vi "Parse rules to postfix.vi"(11 "String":string) -> (3 "Array":T1[](array[typedef]))   [LabVIEW 2019, in "LSS.lvlib"]
doc: "To allow the property control engine to fire events based on multiple conditions, a posfix calculator is used to evaluate the condions. This VI turns the Infix string based by the user to a postfix format that the control engine can read.\n\n<b>Inputs:</b>\n<b>String</b> - Infix string that must be parsed to postfix notation.\n<b>Error In</b> - Standard Error In terminal.\n\n<b>Outputs:</b>\n<b>Postfix</b> - Postfix notation of the input string.\n<b>Error Out</b> - Standard Error out terminal."
uses:
  LSS.lvlib
  Controls/Criteria.ctl
  Controls/Comparison Types.ctl
  <vilib>/regexp/Match Regular Expression.xnode
panel:
  out "Postfix":string[](array[string])
  out "error out":errorcluster
  out "Infix":string[](array[string])
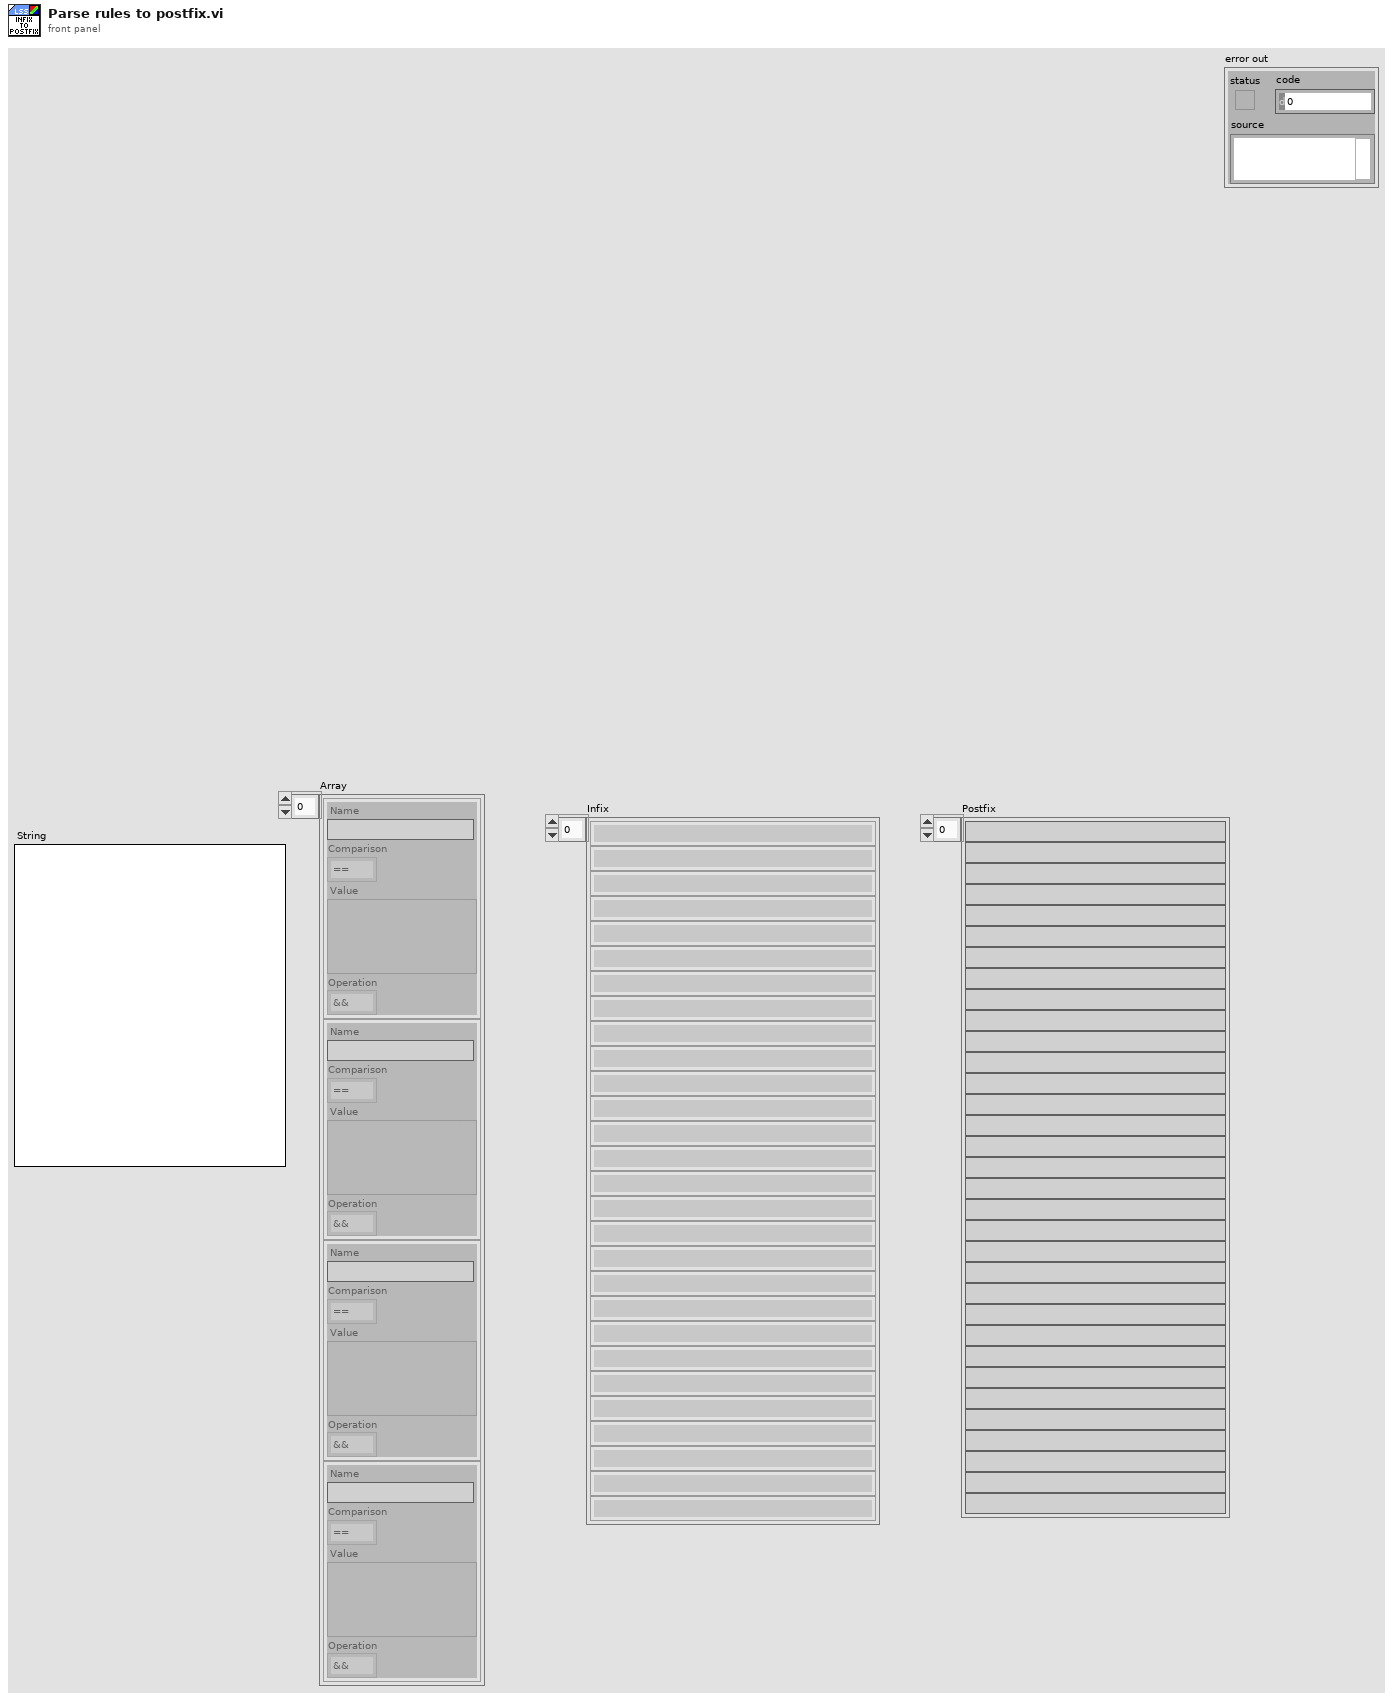
[diagram p1: front panel]
types:
  T1 = typedef "LSS.lvlib/Criteria.ctl" = cluster{"Name":string, "Comparison":T2, "Value":variant, "Operation":enum16{"Stack", "&&", "||"}}
  T2 = typedef "LSS.lvlib/Comparison Types.ctl" = enum16{"==", "!=", "<", ">", "<=", ">="}
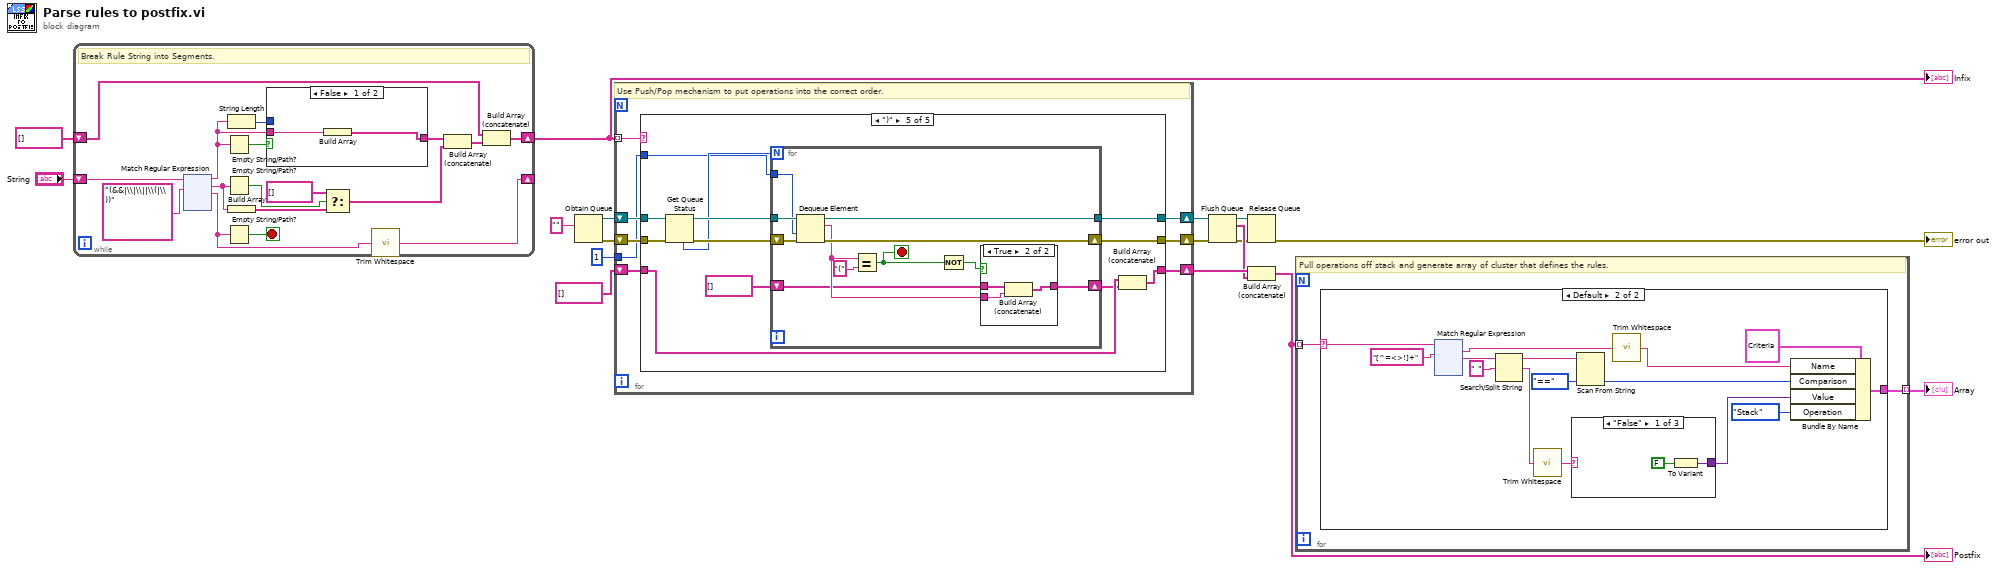
[diagram p0: block diagram]
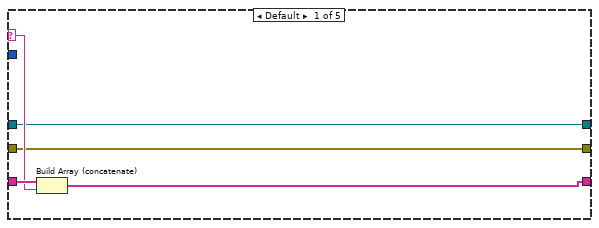
[diagram p2: hidden frame]
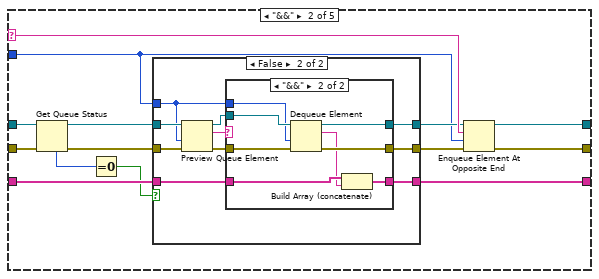
[diagram p3: hidden frame]
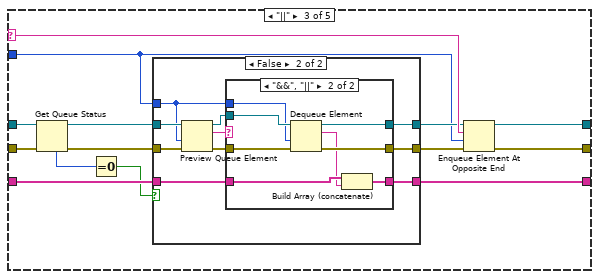
[diagram p6: hidden frame]
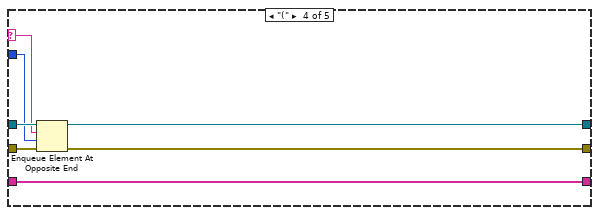
[diagram p9: hidden frame]
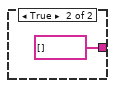
[diagram p11: hidden frame]
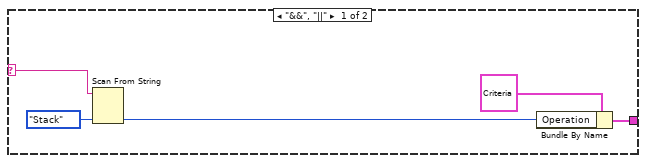
[diagram p12: hidden frame]
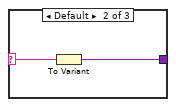
[diagram p13: hidden frame]
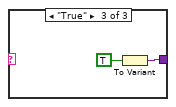
[diagram p14: hidden frame]
diagram:
  n1 = while {
    shift-right: [w18] -> _
    shift-left: "String" -> [w33]
    shift-right: [w20] -> w2
    shift-left: string[] [] -> [w21]
    stop <- w32 stop-if-true
    # "Break Rule String into Segments."
    n2 = xnode "Match Regular Expression"("input string"=w33, "regular expression"="(&&|\\|\\||\\(|\\))") -> ("before match"=w28:string, "whole match"=w23:string, "after match"=w19:string)  [unwired: 4 in, 2 out]
    n3 = Empty String/Path?(string/path=w28) -> (empty?=w31:bool)
    n4 = Empty String/Path?(string/path=w23) -> (empty?=w26:bool)
    n5 = Empty String/Path?(string/path=w19) -> (empty?=w32:bool)
    n6 = String Length(string=w28) -> (length=w30:i32)
    n7 = Build Array(w23) -> (w24:string[])
    n8 = case shown="False" w31 {
      tunnel: w30 -> [_ _]
      tunnel: w28 -> [w36 _]
      tunnel: [w35 string[] []] -> w29
      frame False {
        n9 = Build Array(w36) -> (w35:string[])
      }
      frame True {
      }
    }
    n10 = Select(t=string[] [], s=w26, f=w24) -> (s? t:f=w22:string[])
    n11 = call <vilib>:"Trim Whitespace.vi"("string"=w19) -> ("trimmed string"=w18:string)  [unwired: 1 in]
    n12 = Build Array (concatenate)(w29, w22) -> (w27:string[])
    n13 = Build Array (concatenate)(w21, w27) -> (w20:string[])
  }
  "Infix" <- w2
  n14 = Obtain Queue(element data type="") -> (queue out=w14:refnum<queue>, error out=w13:errorcluster)  [unwired: 4 in, 1 out]
  n15 = for {
    tunnel: w2 -> [w159] mode=indexing
    shift-right: [w156] -> w10
    shift-left: w14 -> [w158]
    shift-right: [w155] -> w9
    shift-left: w13 -> [w157]
    shift-right: [w153] -> w8
    shift-left: string[] [] -> [w154]
    tunnel: 1 -> [w152]
    # "Use Push/Pop mechanism to put operations into the correct order."
    n16 = case shown="\")\"" w159 {
      selector: w159 -> [w163 w176 w214 w242 _]
      tunnel: w158 -> [w161 w175 w213 w247 w259]
      tunnel: w157 -> [w160 w169 w207 w246 w255]
      tunnel: [w161 w178 w216 w245 w257] -> w156
      tunnel: [w160 w177 w215 w244 w258] -> w155
      tunnel: w154 -> [w164 w172 w210 w243 w252]
      tunnel: [w162 w171 w209 w243 w250] -> w153
      tunnel: w152 -> [_ w165 w203 w241 w249]
      frame Default {
        n17 = Build Array (concatenate)(w164, w163) -> (w162:string[])
      }
      frame "&&" {
        n18 = Get Queue Status(queue=w175, error in (no error)=w169) -> (queue out=w170:refnum<queue>, error out=w168:errorcluster, # elements in queue=w166:i32)  [unwired: 1 in, 5 out]
        n19 = Equal To 0?(x=w166) -> (x = 0?=w167:bool)
        n20 = case shown="False" w167 {
          tunnel: w170 -> [w180 w191]
          tunnel: w168 -> [w179 w190]
          tunnel: [w180 w186] -> w174
          tunnel: [w179 w185] -> w173
          tunnel: w172 -> [w181 w184]
          tunnel: [w181 w183] -> w171
          tunnel: w165 -> [_ w182]
          frame True {
          }
          frame False {
            n21 = Preview Queue Element(queue=w191, timeout in ms (-1)=w182, error in (no error)=w190) -> (queue out=w188:refnum<queue>, element=w189:string, error out=w187:errorcluster)  [unwired: 1 out]
            n22 = case shown="\"&&\"" w189 {
              tunnel: w188 -> [w194 w202]
              tunnel: w187 -> [w193 w201]
              tunnel: [w194 w200] -> w186
              tunnel: [w193 w199] -> w185
              tunnel: w184 -> [w192 w198]
              tunnel: [w192 w196] -> w183
              tunnel: w182 -> [_ w195]
              frame Default {
              }
              frame "&&" {
                n23 = Dequeue Element(queue=w202, timeout in ms (-1)=w195, error in (no error)=w201) -> (queue out=w200:refnum<queue>, element=w197:string, error out=w199:errorcluster)  [unwired: 1 out]
                n24 = Build Array (concatenate)(w198, w197) -> (w196:string[])
              }
            }
          }
        }
        n25 = Enqueue Element At Opposite End(queue=w174, element=w176, timeout in ms (-1)=w165, error in (no error)=w173) -> (queue out=w178:refnum<queue>, error out=w177:errorcluster)  [unwired: 1 out]
      }
      frame "||" {
        n26 = Get Queue Status(queue=w213, error in (no error)=w207) -> (queue out=w208:refnum<queue>, error out=w206:errorcluster, # elements in queue=w204:i32)  [unwired: 1 in, 5 out]
        n27 = Equal To 0?(x=w204) -> (x = 0?=w205:bool)
        n28 = case shown="False" w205 {
          tunnel: w208 -> [w218 w229]
          tunnel: w206 -> [w217 w228]
          tunnel: [w218 w224] -> w212
          tunnel: [w217 w223] -> w211
          tunnel: w210 -> [w219 w222]
          tunnel: [w219 w221] -> w209
          tunnel: w203 -> [_ w220]
          frame True {
          }
          frame False {
            n29 = Preview Queue Element(queue=w229, timeout in ms (-1)=w220, error in (no error)=w228) -> (queue out=w226:refnum<queue>, element=w227:string, error out=w225:errorcluster)  [unwired: 1 out]
            n30 = case shown="\"&&\", \"||\"" w227 {
              tunnel: w226 -> [w232 w240]
              tunnel: w225 -> [w231 w239]
              tunnel: [w232 w238] -> w224
              tunnel: [w231 w237] -> w223
              tunnel: w222 -> [w230 w236]
              tunnel: [w230 w234] -> w221
              tunnel: w220 -> [_ w233]
              frame Default {
              }
              frame "&&", "||" {
                n31 = Dequeue Element(queue=w240, timeout in ms (-1)=w233, error in (no error)=w239) -> (queue out=w238:refnum<queue>, element=w235:string, error out=w237:errorcluster)  [unwired: 1 out]
                n32 = Build Array (concatenate)(w236, w235) -> (w234:string[])
              }
            }
          }
        }
        n33 = Enqueue Element At Opposite End(queue=w212, element=w214, timeout in ms (-1)=w203, error in (no error)=w211) -> (queue out=w216:refnum<queue>, error out=w215:errorcluster)  [unwired: 1 out]
      }
      frame "(" {
        n34 = Enqueue Element At Opposite End(queue=w247, element=w242, timeout in ms (-1)=w241, error in (no error)=w246) -> (queue out=w245:refnum<queue>, error out=w244:errorcluster)  [unwired: 1 out]
      }
      frame ")" {
        n35 = Get Queue Status(queue=w259, error in (no error)=w255) -> (queue out=w256:refnum<queue>, error out=w254:errorcluster, # elements in queue=w253:i32)  [unwired: 1 in, 5 out]
        n36 = for {
          N: w253 -> [_]
          tunnel: w256 -> [w270]
          tunnel: [w266] -> w257
          shift-right: [w267] -> w258
          shift-left: w254 -> [w269]
          tunnel: w249 -> [w262]
          shift-right: [w260] -> w251
          shift-left: string[] [] ("Array") -> [w261]
          stop <- w264 stop-if-true
          n37 = Dequeue Element(queue=w270, timeout in ms (-1)=w262, error in (no error)=w269) -> (queue out=w266:refnum<queue>, element=w265:string, error out=w267:errorcluster)  [unwired: 1 out]
          n38 = Equal?(x=w265, y="(") -> (x = y?=w264:bool)
          n39 = Not(x=w264) -> (.not. x?=w263:bool)
          n40 = case shown="True" w263 {
            tunnel: w261 -> [w271 w273]
            tunnel: w265 -> [_ w272]
            tunnel: [w271 w274] -> w260
            frame False {
            }
            frame True {
              n41 = Build Array (concatenate)(w273, w272) -> (w274:string[])
            }
          }
        }
        n42 = Build Array (concatenate)(w252, w251) -> (w250:string[])
      }
    }
  }
  n43 = Flush Queue(queue=w10, error in (no error)=w9) -> (queue out=w6:refnum<queue>, remaining elements=w7:string[], error out=w5:errorcluster)
  n44 = Release Queue(queue=w6, error in (no error)=w5) -> (error out=→"error out":errorcluster)  [unwired: 1 in, 2 out]
  n45 = Build Array (concatenate)(w8, w7) -> (w1:string[])
  "Postfix" <- w1
  n46 = for {
    tunnel: w1 -> [w276] mode=indexing
    tunnel: [w275] -> w17 mode=indexing
    # "Pull operations off stack and generate array of cluster that defines the rules."
    n47 = case shown="Default" w276 {
      selector: w276 -> [w277 w284]
      tunnel: [w280 w283] -> w275
      frame "&&", "||" {
        n48 = Scan From String(input string=w277, default 1=enum16{"Stack", "&&", "||"}."Stack" ("Operation")) -> (output 1=w278:enum16{"Stack", "&&", "||"})  [unwired: 3 in, 3 out]
        n49 = Bundle By Name(cluster=T1 {"Name"="", "Comparison"=enum."==", "Value"=variant, "Operation"=enum."&&"} ("Cluster"), "Operation"=w278) -> (w280:T1)
      }
      frame Default {
        n50 = xnode "Match Regular Expression"("input string"=w284, "regular expression"="[^=<>!]+") -> ("whole match"=w294:string, "after match"=w293:string)  [unwired: 4 in, 3 out]
        n51 = Search/Split String(string=w293, search string/char (-)=" ") -> (substring before match=w291:string, match + rest of string=w288:string)  [unwired: 1 in, 1 out]
        n52 = call <vilib>:"Trim Whitespace.vi"("string"=w288) -> ("trimmed string"=w286:string)  [unwired: 1 in]
        n53 = case shown="\"False\"" w286 {
          selector: w286 -> [_ w300 _]
          tunnel: [w297 w299 w301] -> w285
          frame "False" {
            n54 = To Variant(anything=FALSE) -> (Variant=w297:variant)
          }
          frame Default {
            n55 = To Variant(anything=w300) -> (Variant=w299:variant)
          }
          frame "True" {
            n56 = To Variant(anything=TRUE) -> (Variant=w301:variant)
          }
        }
        n57 = Scan From String(input string=w291, default 1=Comparison_Types."==" ("Comparison")) -> (output 1=w289:T2)  [unwired: 3 in, 3 out]
        n58 = call <vilib>:"Trim Whitespace.vi"("string"=w294) -> ("trimmed string"=w287:string)  [unwired: 1 in]
        n59 = Bundle By Name(cluster=T1 {"Name"="", "Comparison"=enum."==", "Value"=variant, "Operation"=enum."&&"} ("Cluster"), "Name"=w287, "Comparison"=w289, "Value"=w285, "Operation"=enum16{"Stack", "&&", "||"}."Stack") -> (w283:T1)
      }
    }
  }
  "Array" <- w17
